vi "Stimulus.GetStatusInfo.vi"(8 "error in (no error)":errorcluster, 11 "Cluster":T1={"Events.State"=refnum, "Events.Test Result"=refnum, "Events.Progress"=refnum, "INI.Settings"={"Build Location"=path "C:/Simple Sequence Editor/SequenceRepo", "LoggingLocation"=path "", "Sequence.AbortChannel"="", "Sequence.IterationInfoChannel"="", "Sequence.DurationChannel"="", "Sequence.StepInfoChannel"="", "Sequence.SkipChannel"="", "PlotChannels"=[], "Sequence.InitializeScript"=path "C:/Simple Sequence Editor/SequenceRepo", "Sequence.CleanupScript"=path "", "Log.DefaultRate"=0.0}, "NIVS.AlarmManager"=refnum, "NIVS.BaseLogPath"=path "", "NIVS.DataLogManagerRef"=refnum, "NIVS.DataLogSpecRef"=refnum, "NIVS.Deployed"=FALSE, "NIVS.Events"={"SequenceEvent"=refnum, "SystemChangeEvent"=refnum, "WorkspaceEvent"=refnum}, "NIVS.GatewayIPAddress"="", "NIVS.DataLogGUID"="", "NIVS.ProfileCallback"=refnum, "NIVS.ProfileRef"=refnum, "NIVS.SequenceState"=enum."Idle", "NIVS.SystemDefinitionFile"=path "", "NIVS.SystemStateRefs"={"CustDatRef"=refnum, "EvtRef"=refnum, "Target State User Event"=refnum}, "NIVS.WorkspaceManager"=refnum, "NIVS.EventLogGUID"="", "NIVS.EventLogManagerRef"=refnum, "NIVS.EventLogSpecRef"=refnum, "NIVS.BaseToolPath"=path "", "Restart.Path"=path "", "Sequence.#ofColumns"=0, "Sequence.Iterations"=0, "Sequence.Channels"=[], "Sequence.ValidConfig?"=FALSE, "Station.ID"="", "UDP.Queue"=refnum, "UI.Abort"=refnum, "UI.Alarms"=refnum, "UI.Apply"=refnum, "UI.Back"=refnum, "UI.BaseFileName"=refnum, "UI.CurrentIteration"=refnum, "UI.CurrentStep"=refnum, "UI.CyclicFrequency"=refnum, "UI.Description"=refnum, "UI.DelayTime"=refnum, "UI.DisableAlarms"=refnum, "UI.Duration"=refnum, "UI.EnableLogging"=refnum, "UI.EnableState"=refnum, "UI.High"=refnum, "UI.LogChannels"=refnum, "UI.Low"=refnum, "UI.MonitoredVariable"=refnum, "UI.Next"=refnum, "UI.NumberOfCycles"=refnum, "UI.OperatorName"=refnum, "UI.Pause"=refnum, "UI.Profile"=refnum, "UI.Revert"=refnum, "UI.Skip"=refnum, "UI.Start"=refnum, "UI.StartIteration"=refnum, "UI.StartStep"=refnum, "UI.TabControl"=refnum, "UI.TotalIterations"=refnum, "UI.WaveformDefinition"=refnum, "UI.WaveformPreview"=refnum, "UI.WorkOrderNumber"=refnum, "UI.Chart"=refnum, "UI.Status"=refnum, "UI.DataView"=refnum, "UI.Table"=refnum, "UI.Multihead"=refnum, "UI.ToolTab"=refnum, "UI.Result"=refnum, "UI.Log Path"=refnum, "UI.ReportPath"=refnum, "UI.RestartPath"=refnum, "UI.AlarmLog"=refnum}) -> (0 "error out":errorcluster)   [LabVIEW 2015, in "Single Station Execution.lvlib"]
uses:
  Single Station Execution.lvlib
  Types/Main.StateVariables.ctl
  Types/INI.Settings.ctl
  <vilib>/NI Veristand/Execution/AlarmManager/AlarmManagerAPI.ctl
  NationalInstruments.VeriStand.ClientAPI
  <vilib>/NI Veristand/Execution/DataLogging/IDataLogging Ref.ctl
  <vilib>/NI Veristand/Execution/DataLogging/DataLoggingSpecification Ref.ctl
  Types/Execute.UserEventRefs.ctl
  <vilib>/NI Veristand/Execution/Workspace/SystemStateRegEventRef.ctl
  <vilib>/NI Veristand/Execution/Workspace/Target State Info.ctl
  <vilib>/NI Veristand/Execution/Workspace/Target State.ctl
  NationalInstruments.VeriStand.RealTimeSequenceDefinitionApi
  Types/Execution.SequenceState.ctl
  <vilib>/NI Veristand/Execution/Workspace/SystemStateEventRef.ctl
  <vilib>/NI Veristand/Execution/Workspace/WorkspaceAPI.ctl
  Types/UDPEngine.QueueCluster.ctl
  Types/UDPEngine.State.ctl
  <vilib>/NI Veristand/Execution/Workspace/NI VeriStand - Get Single Channel Value.vi
  <vilib>/NI Veristand/Execution/Workspace/NI_VS Workspace ExecutionAPI.lvlib
  <vilib>/NI Veristand/Execution/AlarmManager/NI_VS AlarmManager ExecutionAPI.lvlib
  <vilib>/NI Veristand/Execution/DataLogging/NI_VS Data Logging API.lvlib
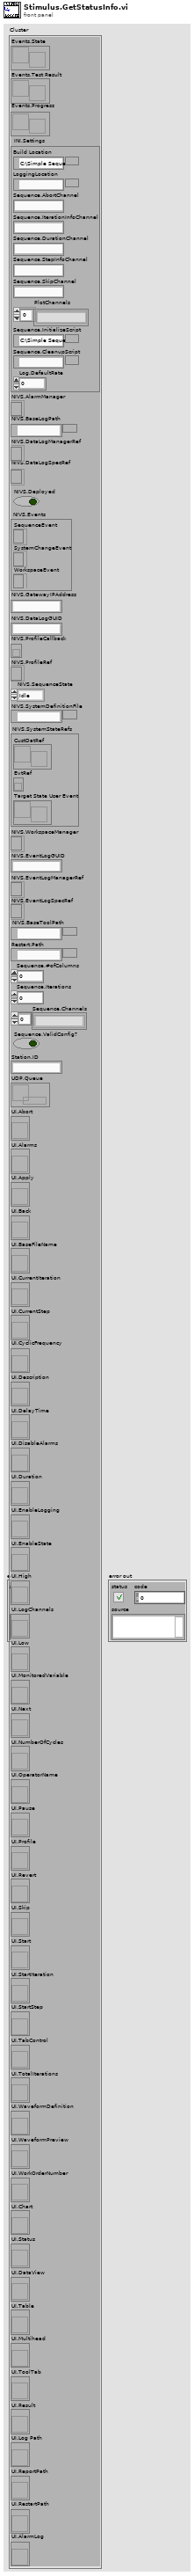
[diagram p1: front panel]
types:
  T1 = typedef "Single Station Execution.lvlib/Main.StateVariables.ctl" = cluster{"Events.State":refnum<user-event>, "Events.Test Result":refnum<user-event>, "Events.Progress":refnum<user-event>, "INI.Settings":T2, "NIVS.AlarmManager":T3, "NIVS.BaseLogPath":path, "NIVS.DataLogManagerRef":T4, "NIVS.DataLogSpecRef":T5, "NIVS.Deployed":bool, "NIVS.Events":T6, "NIVS.GatewayIPAddress":string, "NIVS.DataLogGUID":string, "NIVS.ProfileCallback":refnum<k27>, "NIVS.ProfileRef":refnum<k24>, "NIVS.SequenceState":T8, "NIVS.SystemDefinitionFile":path, "NIVS.SystemStateRefs":T9, "NIVS.WorkspaceManager":T10, "NIVS.EventLogGUID":string, "NIVS.EventLogManagerRef":T4, "NIVS.EventLogSpecRef":T5, "NIVS.BaseToolPath":path, "Restart.Path":path, "Sequence.#ofColumns":i32, "Sequence.Iterations":u32, "Sequence.Channels":string[], "Sequence.ValidConfig?":bool, "Station.ID":string, "UDP.Queue":refnum<queue>, "UI.Abort":refnum<vi>, "UI.Alarms":refnum<vi>, "UI.Apply":refnum<vi>, "UI.Back":refnum<vi>, "UI.BaseFileName":refnum<vi>, "UI.CurrentIteration":refnum<vi>, "UI.CurrentStep":refnum<vi>, "UI.CyclicFrequency":refnum<vi>, "UI.Description":refnum<vi>, "UI.DelayTime":refnum<vi>, "UI.DisableAlarms":refnum<vi>, "UI.Duration":refnum<vi>, "UI.EnableLogging":refnum<vi>, "UI.EnableState":refnum<vi>, "UI.High":refnum<vi>, "UI.LogChannels":refnum<vi>, "UI.Low":refnum<vi>, "UI.MonitoredVariable":refnum<vi>, "UI.Next":refnum<vi>, "UI.NumberOfCycles":refnum<vi>, "UI.OperatorName":refnum<vi>, "UI.Pause":refnum<vi>, "UI.Profile":refnum<vi>, "UI.Revert":refnum<vi>, "UI.Skip":refnum<vi>, "UI.Start":refnum<vi>, "UI.StartIteration":refnum<vi>, "UI.StartStep":refnum<vi>, "UI.TabControl":refnum<vi>, "UI.TotalIterations":refnum<vi>, "UI.WaveformDefinition":refnum<vi>, "UI.WaveformPreview":refnum<vi>, "UI.WorkOrderNumber":refnum<vi>, "UI.Chart":refnum<vi>, "UI.Status":refnum<vi>, "UI.DataView":refnum<vi>, "UI.Table":refnum<vi>, "UI.Multihead":refnum<vi>, "UI.ToolTab":refnum<vi>, "UI.Result":refnum<vi>, "UI.Log Path":refnum<vi>, "UI.ReportPath":refnum<vi>, "UI.RestartPath":refnum<vi>, "UI.AlarmLog":refnum<vi>}
  T2 = typedef "Single Station Execution.lvlib/INI.Settings.ctl" = cluster{"Build Location":path, "LoggingLocation":path, "Sequence.AbortChannel":string, "Sequence.IterationInfoChannel":string, "Sequence.DurationChannel":string, "Sequence.StepInfoChannel":string, "Sequence.SkipChannel":string, "PlotChannels":string[], "Sequence.InitializeScript":path, "Sequence.CleanupScript":path, "Log.DefaultRate":dbl}
  T3 = typedef "NI_VS AlarmManager ExecutionAPI.lvlib/AlarmManagerAPI.ctl" = refnum<k24>
  T4 = typedef "NI_VS Data Logging API.lvlib/IDataLogging Ref.ctl" = refnum<k24>
  T5 = typedef "NI_VS Data Logging API.lvlib/DataLoggingSpecification Ref.ctl" = refnum<k24>
  T6 = typedef "Single Station Execution.lvlib/Execute.UserEventRefs.ctl" = cluster{"SequenceEvent":refnum<event-registration>, "SystemChangeEvent":T7, "WorkspaceEvent":refnum<event-registration>}
  T7 = typedef "NI_VS Workspace ExecutionAPI.lvlib/SystemStateRegEventRef.ctl" = refnum<event-registration>
  T8 = typedef "Single Station Execution.lvlib/Execution.SequenceState.ctl" = enum16{"Idle", "Initializing", "Running", "Paused", "Finalizing", "Complete"}
  T9 = typedef "NI_VS Workspace ExecutionAPI.lvlib/SystemStateEventRef.ctl" = cluster{"CustDatRef":refnum<user-event>, "EvtRef":refnum<k27>, "Target State User Event":refnum<user-event>}
  T10 = typedef "NI_VS Workspace ExecutionAPI.lvlib/WorkspaceAPI.ctl" = refnum<k24>
  T11 = enum16{"Disabled", "Enabled", "Tripped", "Delayed Trip", "Indicate"}
  T12 = typedef "NI_VS Alarm ExecutionAPI.lvlib/AlarmInfo.ctl" = cluster{"Watch Channel":string, "High Limit Constant":bool, "High Limit Channel":string, "High Limit":dbl, "Low Limit Constant":bool, "Low Limit Channel":string, "Low Limit":dbl, "Procedure Name":string, "Delay":dbl, "Trip Value":dbl, "Priority":enum16{"Low", "Medium", "High"}, "State":enum16{"Disabled", "Enabled", "Tripped", "Delayed Trip", "Indicate"}, "Mode":enum16{"Normal", "Indicate Only"}, "Group Number":u32, "Priority Number":u32, "Name":string, "Full Name":string}
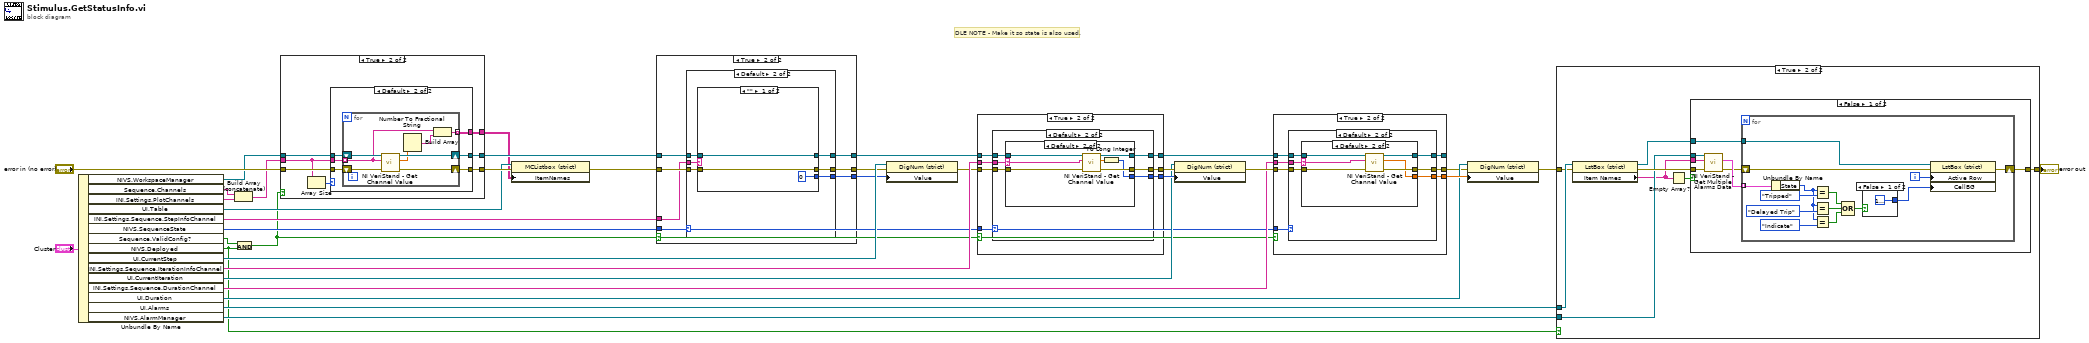
[diagram p0: block diagram]
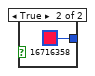
[diagram p5: hidden frame]
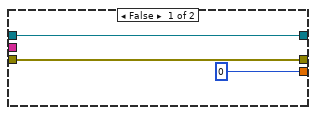
[diagram p7: hidden frame]
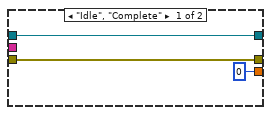
[diagram p8: hidden frame]
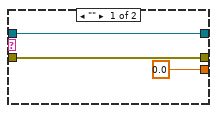
[diagram p9: hidden frame]
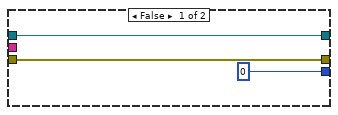
[diagram p10: hidden frame]
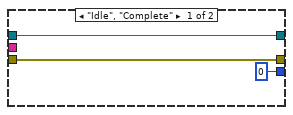
[diagram p11: hidden frame]
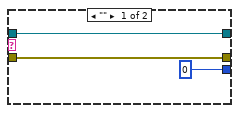
[diagram p12: hidden frame]
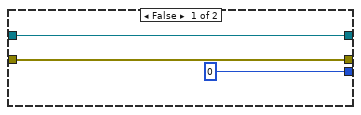
[diagram p13: hidden frame]
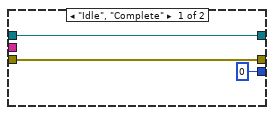
[diagram p14: hidden frame]
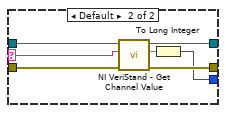
[diagram p15: hidden frame]
diagram:
  # "DLE NOTE - Make it so state is also used."
  n1 = Unbundle By Name("Cluster") -> ("NIVS.WorkspaceManager"=w12:T10, "Sequence.Channels"=w5:string[], "INI.Settings.PlotChannels"=w6:string[], "UI.Table"=w8:refnum<vi>, "INI.Settings.Sequence.StepInfoChannel"=w33:string, "NIVS.SequenceState"=w19:T8, "Sequence.ValidConfig?"=w3:bool, "NIVS.Deployed"=w2:bool, "UI.CurrentStep"=w31:refnum<vi>, "INI.Settings.Sequence.IterationInfoChannel"=w35:string, "UI.CurrentIteration"=w27:refnum<vi>, "INI.Settings.Sequence.DurationChannel"=w24:string, "UI.Duration"=w22:refnum<vi>, "UI.Alarms"=w17:refnum<vi>, "NIVS.AlarmManager"=w16:T3)
  n2 = Build Array (concatenate)(w5, w6) -> (w4:string[])
  n3 = And(x=w3, y=w2) -> (x .and. y?=w1:bool)
  n4 = case shown="True" w1 {
    tunnel: w12 -> [w36 w42]
    tunnel: "error in (no error)" -> [w37 w44]
    tunnel: [w37 w43] -> w10
    tunnel: w4 -> [_ w39]
    tunnel: [w36 w41] -> w11
    tunnel: [_ w38] -> w7
    frame False {
    }
    frame True {
      n5 = Array Size(array=w39) -> (size(s)=w40:i32)
      n6 = case shown="Default" w40 {
        tunnel: w44 -> [w46 w52]
        tunnel: [w46 w51] -> w43
        tunnel: w42 -> [w45 w50]
        tunnel: [w45 w49] -> w41
        tunnel: w39 -> [_ w48]
        tunnel: [_ w47] -> w38
        frame 0 {
        }
        frame Default {
          n7 = for {
            tunnel: w48 -> [w54] mode=indexing
            shift-right: [w59] -> w51
            shift-left: w52 -> [w60]
            shift-right: [w57] -> w49
            shift-left: w50 -> [w58]
            tunnel: [w53] -> w47 mode=indexing
            n8 = call-poly <vilib>:"NI VeriStand - Get Channel Value.vi"("error in (no error)"=w60, "Channel"=w54, "WorkspaceManager in"=w58) -> ("error out"=w59:errorcluster, "Value"=w56:dbl, "WorkspaceManager out"=w57:T10)  [unwired: 6 in]
            n9 = Number To Fractional String(number=w56) -> (F-format string=w55:string)  [unwired: 3 in]
            n10 = Build Array(w54, w55) -> (w53:string[])
          }
        }
      }
    }
  }
  n11 = property class="MCListbox (strict)"(reference=w8, error in=w10, "ItemNames"=w7) -> (error out=w9:errorcluster)  [unwired: 1 out]
  n12 = case shown="True" w1 {
    tunnel: w11 -> [w61 w68]
    tunnel: w9 -> [w63 w70]
    tunnel: [w63 w69] -> w30
    tunnel: w33 -> [_ w66]
    tunnel: [0 w67] -> w20
    tunnel: [w61 w65] -> w34
    tunnel: w19 -> [_ w64]
    frame False {
    }
    frame True {
      n13 = case shown="Default" w64 {
        tunnel: w70 -> [w72 w79]
        tunnel: [w72 w78] -> w69
        tunnel: w68 -> [w73 w77]
        tunnel: [0 w76] -> w67
        tunnel: w66 -> [_ w75]
        tunnel: [w73 w74] -> w65
        frame "Idle", "Complete" {
        }
        frame Default {
          n14 = case shown="\"\"" w75 {
            selector: w75 -> [_ w83]
            tunnel: w79 -> [w82 w89]
            tunnel: [w82 w88] -> w78
            tunnel: w77 -> [w80 w87]
            tunnel: [0 w85] -> w76
            tunnel: [w80 w84] -> w74
            frame "" {
            }
            frame Default {
              n15 = call-poly <vilib>:"NI VeriStand - Get Channel Value.vi"("error in (no error)"=w89, "Channel"=w83, "WorkspaceManager in"=w87) -> ("error out"=w88:errorcluster, "Value"=w86:dbl, "WorkspaceManager out"=w84:T10)  [unwired: 6 in]
              n16 = To Long Integer(number=w86) -> (32bit integer=w85:i32)
            }
          }
        }
      }
    }
  }
  n17 = property class="DigNum (strict)"(reference=w31, error in=w30, "Value"=w20) -> (error out=w21:errorcluster)  [unwired: 1 out]
  n18 = case shown="True" w1 {
    tunnel: w34 -> [w90 w97]
    tunnel: w21 -> [w92 w99]
    tunnel: [w92 w98] -> w29
    tunnel: w35 -> [_ w95]
    tunnel: [0 w96] -> w28
    tunnel: w19 -> [_ w94]
    tunnel: [w90 w93] -> w23
    frame False {
    }
    frame True {
      n19 = case shown="Default" w94 {
        tunnel: w99 -> [w102 w108]
        tunnel: [w102 w107] -> w98
        tunnel: w97 -> [w100 w106]
        tunnel: [0 w105] -> w96
        tunnel: w95 -> [_ w104]
        tunnel: [w100 w103] -> w93
        frame "Idle", "Complete" {
        }
        frame Default {
          n20 = case shown="Default" w104 {
            selector: w104 -> [_ w112]
            tunnel: w108 -> [w111 w118]
            tunnel: [w111 w117] -> w107
            tunnel: w106 -> [w109 w116]
            tunnel: [0 w114] -> w105
            tunnel: [w109 w113] -> w103
            frame "" {
            }
            frame Default {
              n21 = call-poly <vilib>:"NI VeriStand - Get Channel Value.vi"("error in (no error)"=w118, "Channel"=w112, "WorkspaceManager in"=w116) -> ("error out"=w117:errorcluster, "Value"=w115:dbl, "WorkspaceManager out"=w113:T10)  [unwired: 6 in]
              n22 = To Long Integer(number=w115) -> (32bit integer=w114:i32)
            }
          }
        }
      }
    }
  }
  n23 = property class="DigNum (strict)"(reference=w27, error in=w29, "Value"=w28) -> (error out=w26:errorcluster)  [unwired: 1 out]
  n24 = case shown="True" w1 {
    tunnel: w23 -> [w119 w126]
    tunnel: w26 -> [w121 w128]
    tunnel: [w121 w127] -> w18
    tunnel: w24 -> [_ w124]
    tunnel: [0 w125] -> w25
    tunnel: w19 -> [_ w123]
    tunnel: [w119 w122] -> _
    frame False {
    }
    frame True {
      n25 = case shown="Default" w123 {
        tunnel: w128 -> [w131 w137]
        tunnel: [w131 w136] -> w127
        tunnel: w126 -> [w129 w135]
        tunnel: [0 w134] -> w125
        tunnel: w124 -> [_ w133]
        tunnel: [w129 w132] -> w122
        frame "Idle", "Complete" {
        }
        frame Default {
          n26 = case shown="Default" w133 {
            selector: w133 -> [_ w141]
            tunnel: w137 -> [w140 w146]
            tunnel: [w140 w145] -> w136
            tunnel: w135 -> [w138 w144]
            tunnel: [0.0 w142] -> w134
            tunnel: [w138 w143] -> w132
            frame "" {
            }
            frame Default {
              n27 = call-poly <vilib>:"NI VeriStand - Get Channel Value.vi"("error in (no error)"=w146, "Channel"=w141, "WorkspaceManager in"=w144) -> ("error out"=w145:errorcluster, "Value"=w142:dbl, "WorkspaceManager out"=w143:T10)  [unwired: 6 in]
            }
          }
        }
      }
    }
  }
  n28 = property class="DigNum (strict)"(reference=w22, error in=w18, "Value"=w25) -> (error out=w15:errorcluster)  [unwired: 1 out]
  n29 = case shown="True" w2 {
    tunnel: w17 -> [_ w155]
    tunnel: w16 -> [_ w153]
    tunnel: w15 -> [w147 w151]
    tunnel: [w147 w150] -> w14
    frame False {
    }
    frame True {
      n30 = property class="LstBox (strict)"(reference=w155, error in=w151) -> (reference out=w152:refnum<vi>, error out=w154:errorcluster, "Item Names"=w149:string[])
      n31 = Empty Array?(array=w149) -> (empty?=w148:bool)
      n32 = case shown="False" w148 {
        tunnel: w154 -> [w162 w179]
        tunnel: w153 -> [w161 _]
        tunnel: w152 -> [w159 _]
        tunnel: [w157 w179] -> w150
        tunnel: w149 -> [w156 _]
        frame False {
          n33 = call <vilib>:"NI VeriStand - Get Multiple Alarms Data.vi"("error in (no error)"=w162, "Alarm Names"=w156, "AlarmManager in"=w161) -> ("error out"=w158:errorcluster, "Alarms Data"=w160:T12[])  [unwired: 6 in, 1 out]
          n34 = for {
            tunnel: w160 -> [w176] mode=indexing
            tunnel: w159 -> [w168]
            shift-right: [w163] -> w157
            shift-left: w158 -> [w164]
            i -> [w167]
            n35 = Unbundle By Name(w176) -> ("State"=w172:T11)
            n36 = Equal?(x=w172, y=T11."Tripped") -> (x = y?=w171:bool)
            n37 = Equal?(x=w172, y=T11."Delayed Trip") -> (x = y?=w170:bool)
            n38 = Equal?(x=w172, y=T11."Indicate") -> (x = y?=w169:bool)
            n39 = Compound Arithmetic op=OR(w171, w170, w169) -> (w165:bool)
            n40 = case shown="False" w165 {
              tunnel: [u32 16777216 u32 16716358] -> w166
              frame False {
              }
              frame True {
              }
            }
            n41 = property class="LstBox (strict)"(reference=w168, error in=w164, "Active Row"=w167, "CellBG"=w166) -> (error out=w163:errorcluster)  [unwired: 1 out]
          }
        }
        frame True {
        }
      }
    }
  }
  "error out" <- w14
